vi "Shift Register - Tank Filling with Average of Last 5 Readings.vi"() -> ()   [LabVIEW 2016]
panel:
  out "Average":i32
  out "Numeric 1":i32
  out "Tank":dbl(slide) scale=0.0..100.0
  in  "Input":i32
  out "Tank Level":i32
  out "Numeric 4":i32
  out "Numeric 3":i32
  out "Numeric 2":i32
  out "Numeric 5":i32
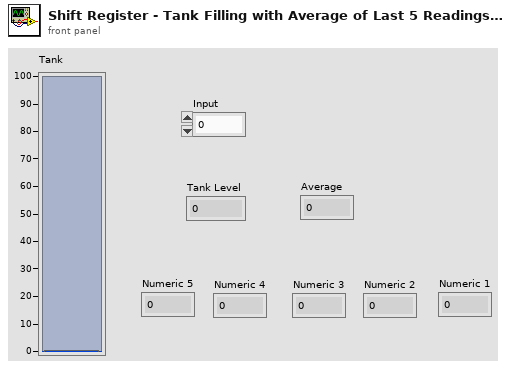
[diagram p1: front panel]
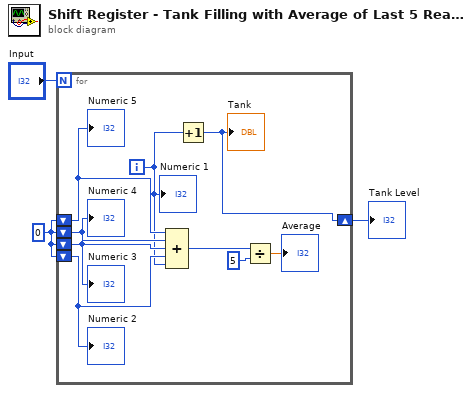
[diagram p0: block diagram]
diagram:
  w1 = 0
  n1 = for {
    N: "Input" -> [_]
    shift-right: [w12] -> w3
    shift-left: w1 -> [w9]
    shift-left: w1 -> [w8]
    shift-left: w1 -> [w7]
    shift-left: w1 -> [w6]
    i -> [w4]
    n2 = Compound Arithmetic op=ADD(w9, w8, w7, w6, w4) -> (w5:i32)
    n3 = Increment(x=w4) -> (x+1=w12:i32)
    "Tank" <- w12
    n4 = Divide(x=w5, y=5) -> (x/y=→"Average":dbl)
    "Numeric 4" <- w8
    "Numeric 3" <- w7
    "Numeric 2" <- w6
    "Numeric 5" <- w9
    "Numeric 1" <- w4
  }
  "Tank Level" <- w3
